vi "PID.vi"() -> ()   [LabVIEW 2020]
uses:
  <vilib>/Instr/_visa.llb/VISA Configure Serial Port (Instr).vi
panel:
  in  "VISA resource":refnum<visa-resource-name>="COM4"
  in  "Stop":bool
  out "SP and PV":cluster{"initial PV":dbl, "SP1:":dbl}(graph)={"initial PV"=50.98160323470328, "SP1:"=50.98039215686275}
  in  "PID Gains":cluster{"Kp":dbl, "Ki":dbl, "Kd":dbl}={"Kp"=2.5, "Ki"=0.02, "Kd"=0.0} {"Kd" format="%#.6g"; "Ki" format="%#.6g"; "Kp" format="%#.6g"}
  in  "SP:":dbl(slide)=50.98039215686275 min=0.0 max=0.0 scale=0.0..300.0
  out "PV:":dbl(slide)=50.98160323470328 scale=0.0..300.0
  out "remain\nvalue":string
  out "before\ntemp":string
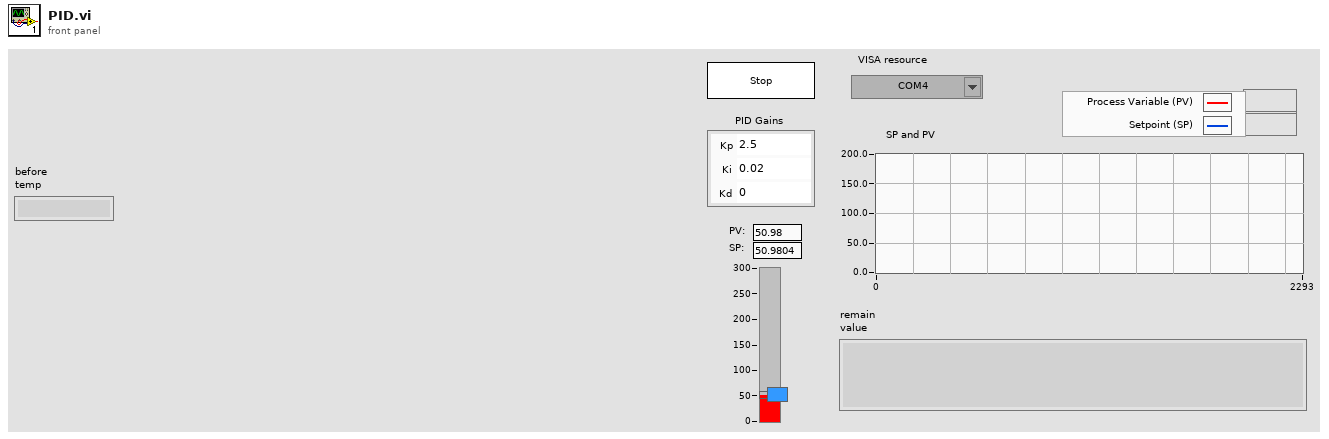
[diagram p1: front panel]
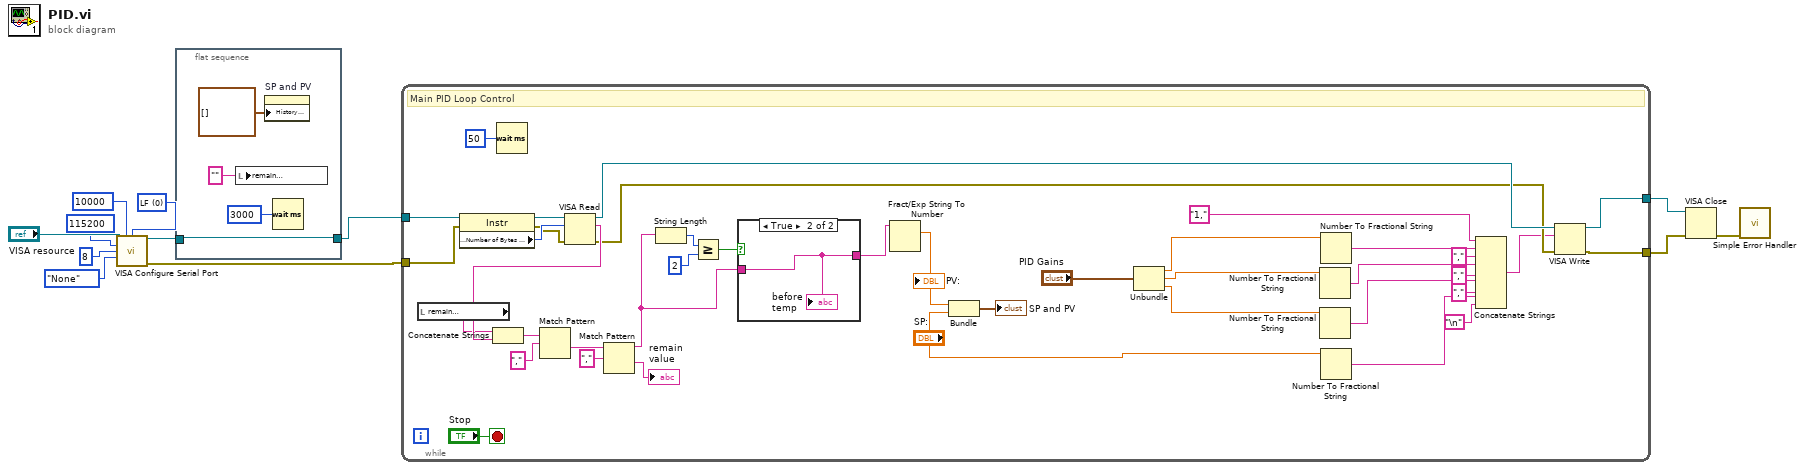
[diagram p0: block diagram]
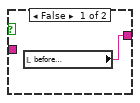
[diagram p2: hidden frame]
diagram:
  w9 = u16 0 items=["LF"]
  n1 = call-poly "VISA Configure Serial Port"("VISA resource name"="VISA resource", "timeout (10sec)"=u32 10000, "termination char\n(0xA = '\\n' = LF)"=w9, "baud rate (9600)"=u32 115200, "data bits (8)"=u16 8, "parity (0:none)"=enum16{"None", "Odd", "Even", "Mark", "Space"}."None") -> ("VISA resource name out"=w11:refnum<visa-resource-name>, "error out"=w1:errorcluster)  [unwired: 8 in]
  n2 = flat-sequence {
    tunnel: [w15] -> w2
    tunnel: w11 -> [w15]
    frame #0 {
      n3 = local write "remain\nvalue"("" ("after substring")) -> ()
      n4 = property on="SP and PV" class="WFChart (strict)"("History Data"=cluster{"initial PV":dbl, "SP1:":dbl}[] []) -> ()  [unwired: 2 in, 2 out]
      n5 = Wait (ms)(milliseconds to wait=u32 3000 ("대기 시간(ms)")) -> ()  [unwired: 1 out]
    }
  }
  n6 = while {
    tunnel: w1 -> [w51]
    tunnel: w2 -> [w50]
    tunnel: [w33] -> w4
    tunnel: [w31] -> w3
    stop <- "Stop" stop-if-true
    # "Main PID Loop Control"
    n7 = local read "remain\nvalue"() -> (w41:string)
    n8 = property class="Instr"(reference=w50, error in=w51) -> (reference out=w52:refnum<visa-resource-name>, error out=w48:errorcluster, "Serial Settings:Number of Bytes at Serial Port"=w49:u32)
    n9 = Wait (ms)(milliseconds to wait=u32 50 ("대기 시간(ms)")) -> ()  [unwired: 1 out]
    n10 = VISA Read(VISA resource name=w52, byte count=w49, error in (no error)=w48) -> (VISA resource name out=w34:refnum<visa-resource-name>, read buffer=w42:string, error out=w32:errorcluster)  [unwired: 1 out]
    n11 = Concatenate Strings(w41, w42) -> (w46:string)
    n12 = Match Pattern(string=w46, regular expression=",") -> (after substring=w45:string)  [unwired: 1 in, 3 out]
    n13 = Match Pattern(string=w45, regular expression=",") -> (before substring=w36:string, after substring=→"remain\nvalue":string)  [unwired: 1 in, 2 out]
    n14 = String Length(string=w36) -> (length=w39:i32)
    n15 = Greater Or Equal?(x=w39, y=2) -> (x >= y?=w38:bool)
    n16 = case shown="True" w38 {
      tunnel: [w57 w58] -> w35
      tunnel: w36 -> [_ w58]
      frame False {
        n17 = local read "before\ntemp"() -> (w57:string)
      }
      frame True {
        "before\ntemp" <- w58
      }
    }
    n18 = Fract/Exp String To Number(string=w35) -> (number=w30:dbl)  [unwired: 3 in, 1 out]
    "PV:" <- w30
    n19 = Bundle(w30, "SP:"="SP:") -> (→"SP and PV":cluster{dbl, "SP:":dbl})  [unwired: 1 in]
    n20 = Unbundle("PID Gains") -> ("Kp"=w19:dbl, "Ki"=w18:dbl, "Kd"=w17:dbl)
    n21 = Number To Fractional String(number=w18) -> (F-format string=w22:string)  [unwired: 3 in]
    n22 = Number To Fractional String(number=w17) -> (F-format string=w21:string)  [unwired: 3 in]
    n23 = Number To Fractional String(number=w19) -> (F-format string=w20:string)  [unwired: 3 in]
    n24 = Number To Fractional String(number="SP:") -> (F-format string=w24:string)  [unwired: 3 in]
    n25 = Concatenate Strings("1,", w20, "," ("string"), w22, "," ("string"), w21, "," ("string"), w24, "\n") -> (w29:string)
    n26 = VISA Write(VISA resource name=w34, write buffer=w29, error in (no error)=w32) -> (VISA resource name out=w33:refnum<visa-resource-name>, error out=w31:errorcluster)  [unwired: 1 out]
  }
  n27 = VISA Close(VISA resource name=w4, error in (no error)=w3) -> (error out=w5:errorcluster)
  n28 = call <vilib>:"Simple Error Handler.vi"("error in (no error)"=w5) -> ()  [unwired: 4 in, 5 out]
